vi "FGV - Pattern Name.vi"(1 "String":string, 2 "Operation":T1) -> (0 "String out":string)   [LabVIEW 2018, in "File Parser Interface.lvlib" / "File Parser Interface.lvclass"]
uses:
  File Parser Interface.lvclass
  Operations - FGV.ctl
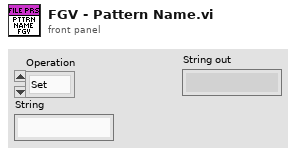
[diagram p1: front panel]
types:
  T1 = typedef "File Parser Interface.lvlib/File Parser Interface.lvclass/Operations - FGV.ctl" = enum16{"Set", "Get", "Clear"}
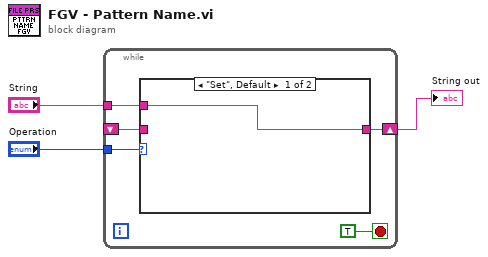
[diagram p0: block diagram]
diagram:
  n1 = while {
    tunnel: "Operation" -> [w7]
    tunnel: "String" -> [w6]
    shift-right: [w5] -> w1
    shift-left: _ -> [w4]
    stop <- TRUE stop-if-true
    n2 = case shown="\"Set\", Default" w7 {
      tunnel: w6 -> [w9 _]
      tunnel: [w9 w10] -> w5
      tunnel: w4 -> [_ w10]
      frame "Set", Default {
      }
      frame "Get" {
      }
    }
  }
  "String out" <- w1
